vi "ZyklussteuerungGV_ECD.vi"(0 "Traps/MachKoeff0":dbl[](array[numeric]), 1 "DIOsNummern":cluster{"DIOsMod2BNr":i32[]}[](array[cluster]), 2 "error in":errorcluster, 5 "Traps/MachKoeff1":dbl[](array[numeric]), 7 "FPGA-VI-Referenz":refnum<k20>, 9 "Traps/MachKoeff2":dbl[](array[numeric]), 11 "Schieberegister":T1, 12 "Zeitpunkte/Setpoints":T2) -> (4 "Schieberegister":T1, 8 "error out":errorcluster)   [LabVIEW 2017]
uses:
  GVZwangs.vi
  GVHeizenLH.vi
  GVZeitenZyklen.vi
  <vilib>/Utility/error.llb/Error Cluster From Error Code.vi
  <vilib>/rvi/errors/niLvFpgaAdjustHostInterfaceError.vi
  GVHorstSP.vi
  GVZwangsMPV.vi
  GVZwangsMPVPos.vi
  GVVentilposition.vi
  <vilib>/rvi/interface/nirviReadWriteControl/nirviReadWriteControl.xnode
  FPGA Bitfiles/HAGAR-VECD_FPGATarget_FPGA-ProgrammECD_WS++LmW9gGg.lvbitx
  FPGA-Programm_ECD.vi
  NiFpgaLv.dll
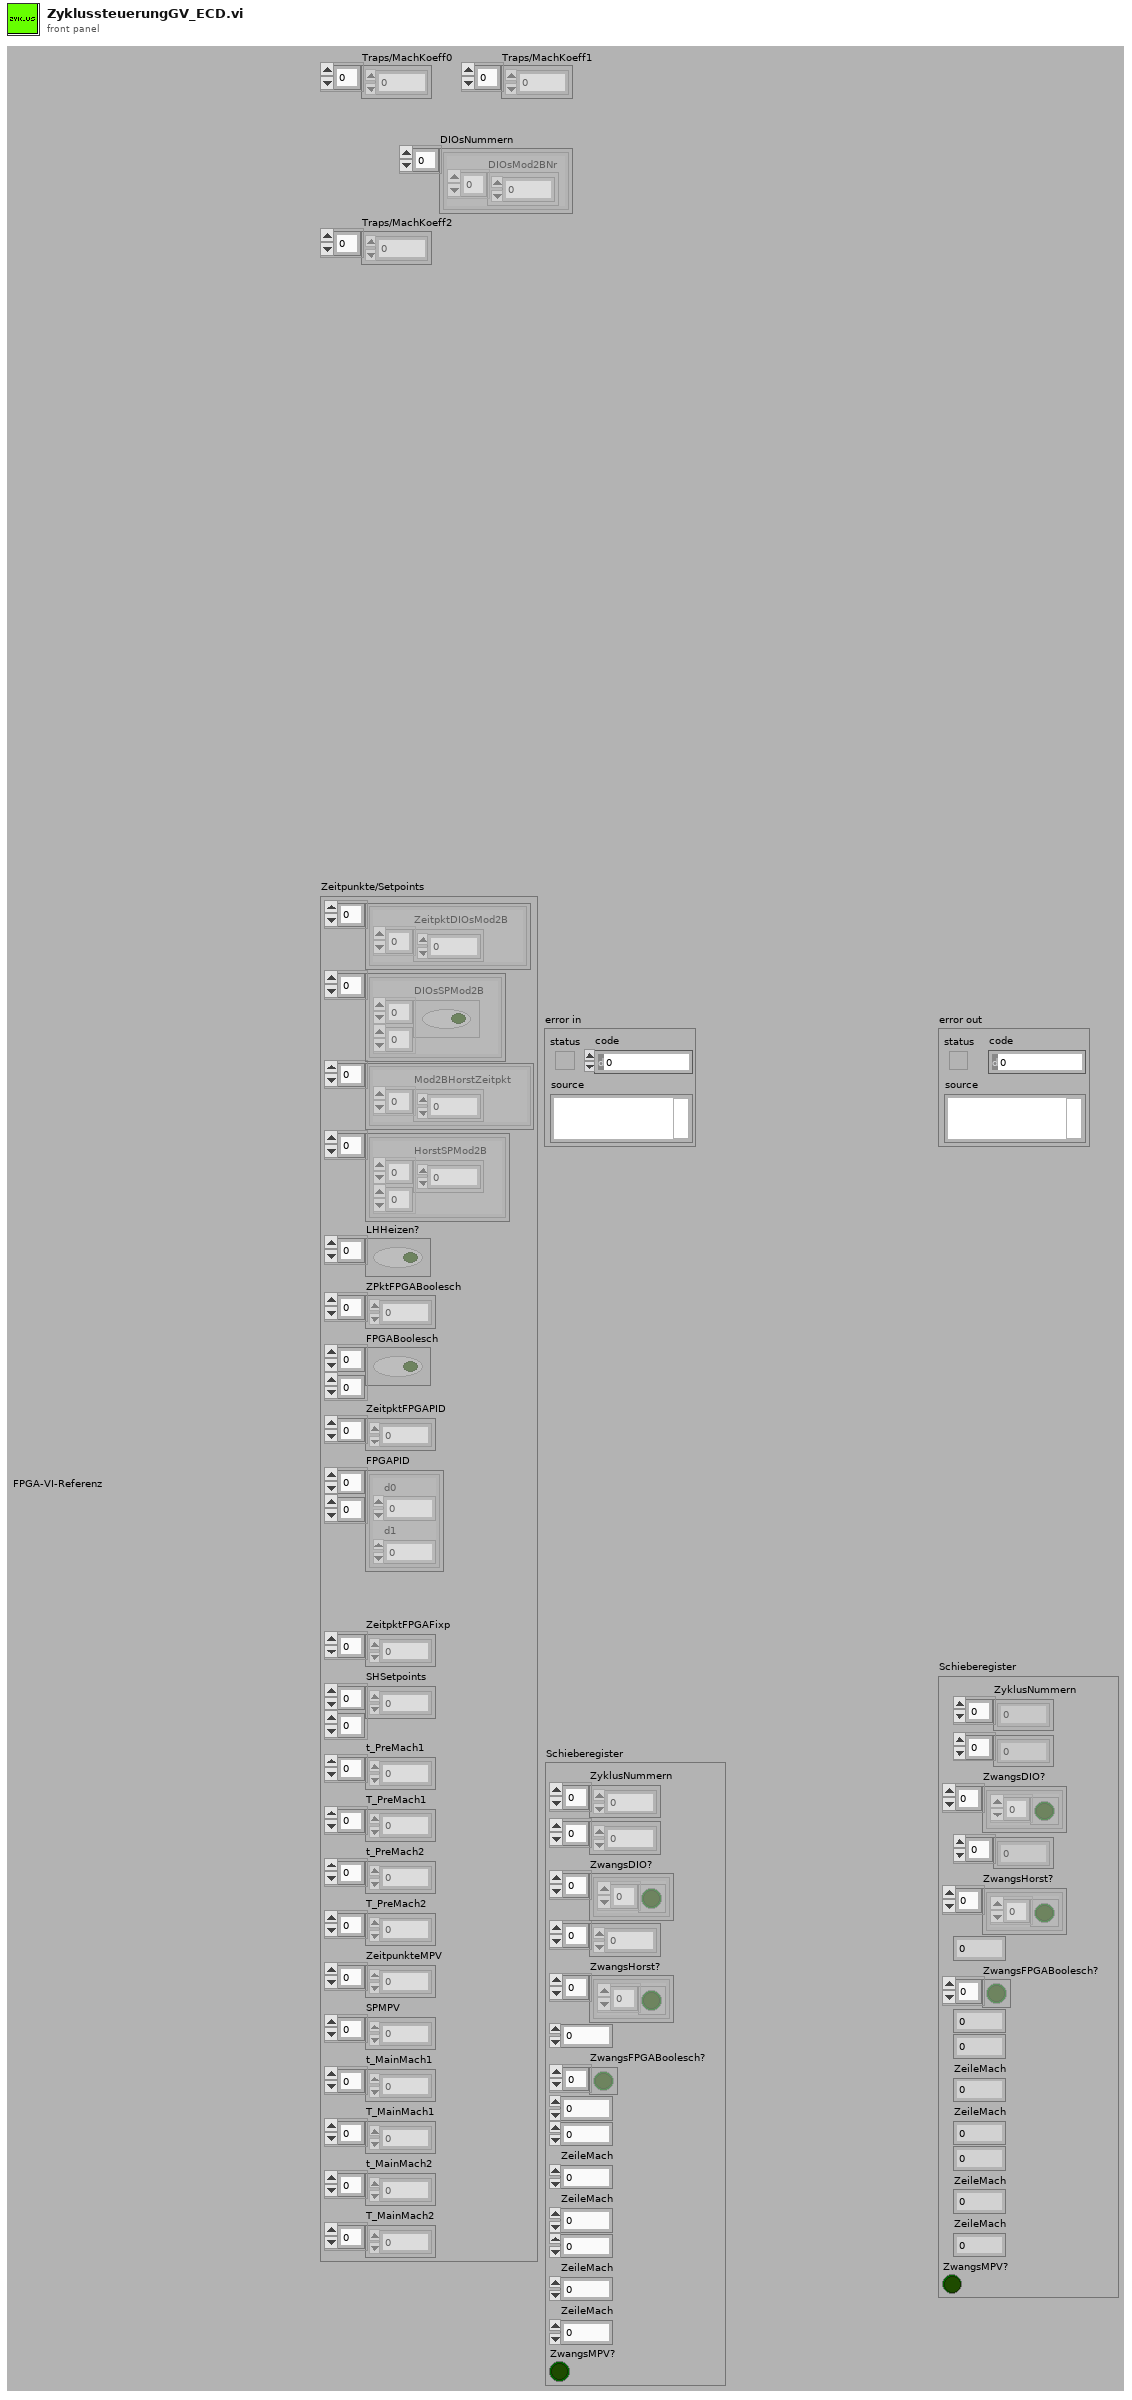
[diagram p1: front panel]
types:
  T1 = cluster{"ZyklusNummern":i32[], i32[], "ZwangsDIO?":cluster{bool[]}[], i32[], "ZwangsHorst?":cluster{bool[]}[], i32, "ZwangsFPGABoolesch?":bool[], i32, i32, "ZeileMach":i32, "ZeileMach":i32, i32, "ZeileMach":i32, "ZeileMach":i32, "ZwangsMPV?":bool}
  T2 = cluster{cluster{"ZeitpktDIOsMod2B":dbl[]}[], cluster{"DIOsSPMod2B":bool[][]}[], cluster{"Mod2BHorstZeitpkt":dbl[]}[], cluster{"HorstSPMod2B":dbl[][]}[], "LHHeizen?":bool[], "ZPktFPGABoolesch":dbl[], "FPGABoolesch":bool[][], "ZeitpktFPGAPID":dbl[], "FPGAPID":cluster{"d0":fxp<+/-,18,18>, "d1":fxp<+/-,21,21>}[][], "ZeitpktFPGAFixp":dbl[], "SHSetpoints":dbl[][], "t_PreMach1":dbl[], "T_PreMach1":dbl[], "t_PreMach2":dbl[], "T_PreMach2":dbl[], "ZeitpunkteMPV":dbl[], "SPMPV":i32[], "t_MainMach1":dbl[], "T_MainMach1":dbl[], "t_MainMach2":dbl[], "T_MainMach2":dbl[]}
  T3 = cluster{"d0":fxp<+/-,18,18>, "d1":fxp<+/-,21,21>}[][]
  T4 = cluster{"[0]":bool, "[1]":bool, "[2]":bool, "[3]":bool, "[4]":bool, "[5]":bool, "[6]":bool, "[7]":bool, "[8]":bool, "[9]":bool, "[10]":bool, "[11]":bool, "[12]":bool, "[13]":bool, "[14]":bool, "[15]":bool, "[16]":bool, "[17]":bool, "[18]":bool, "[19]":bool, "[20]":bool, "[21]":bool, "[22]":bool, "[23]":bool, "[24]":bool, "[25]":bool, "[26]":bool, "[27]":bool, "[28]":bool, "[29]":bool, "[30]":bool, "[31]":bool}
  T5 = cluster{"[0]":bool, "[1]":bool, "[2]":bool, "[3]":bool, "[4]":bool, "[5]":bool}
  T6 = cluster{"d0":fxp<+/-,18,18>, "d1":fxp<+/-,21,21>}[]
  T7 = cluster{"FPGAPID[0]":cluster{"d0":fxp<+/-,18,18>, "d1":fxp<+/-,21,21>}, "FPGAPID[1]":cluster{"d0":fxp<+/-,18,18>, "d1":fxp<+/-,21,21>}, "FPGAPID[2]":cluster{"d0":fxp<+/-,18,18>, "d1":fxp<+/-,21,21>}, "FPGAPID[3]":cluster{"d0":fxp<+/-,18,18>, "d1":fxp<+/-,21,21>}, "FPGAPID[4]":cluster{"d0":fxp<+/-,18,18>, "d1":fxp<+/-,21,21>}, "FPGAPID[5]":cluster{"d0":fxp<+/-,18,18>, "d1":fxp<+/-,21,21>}}
  T8 = cluster{"d0":fxp<+/-,18,18>, "d1":fxp<+/-,21,21>}
  T9 = cluster{"setpoint":fxp<+/-,26,5>, "setpoint":fxp<+/-,26,5>, "[2]":fxp<+/-,26,5>, "[3]":fxp<+/-,26,5>, "[4]":fxp<+/-,26,5>, "[5]":fxp<+/-,26,5>}
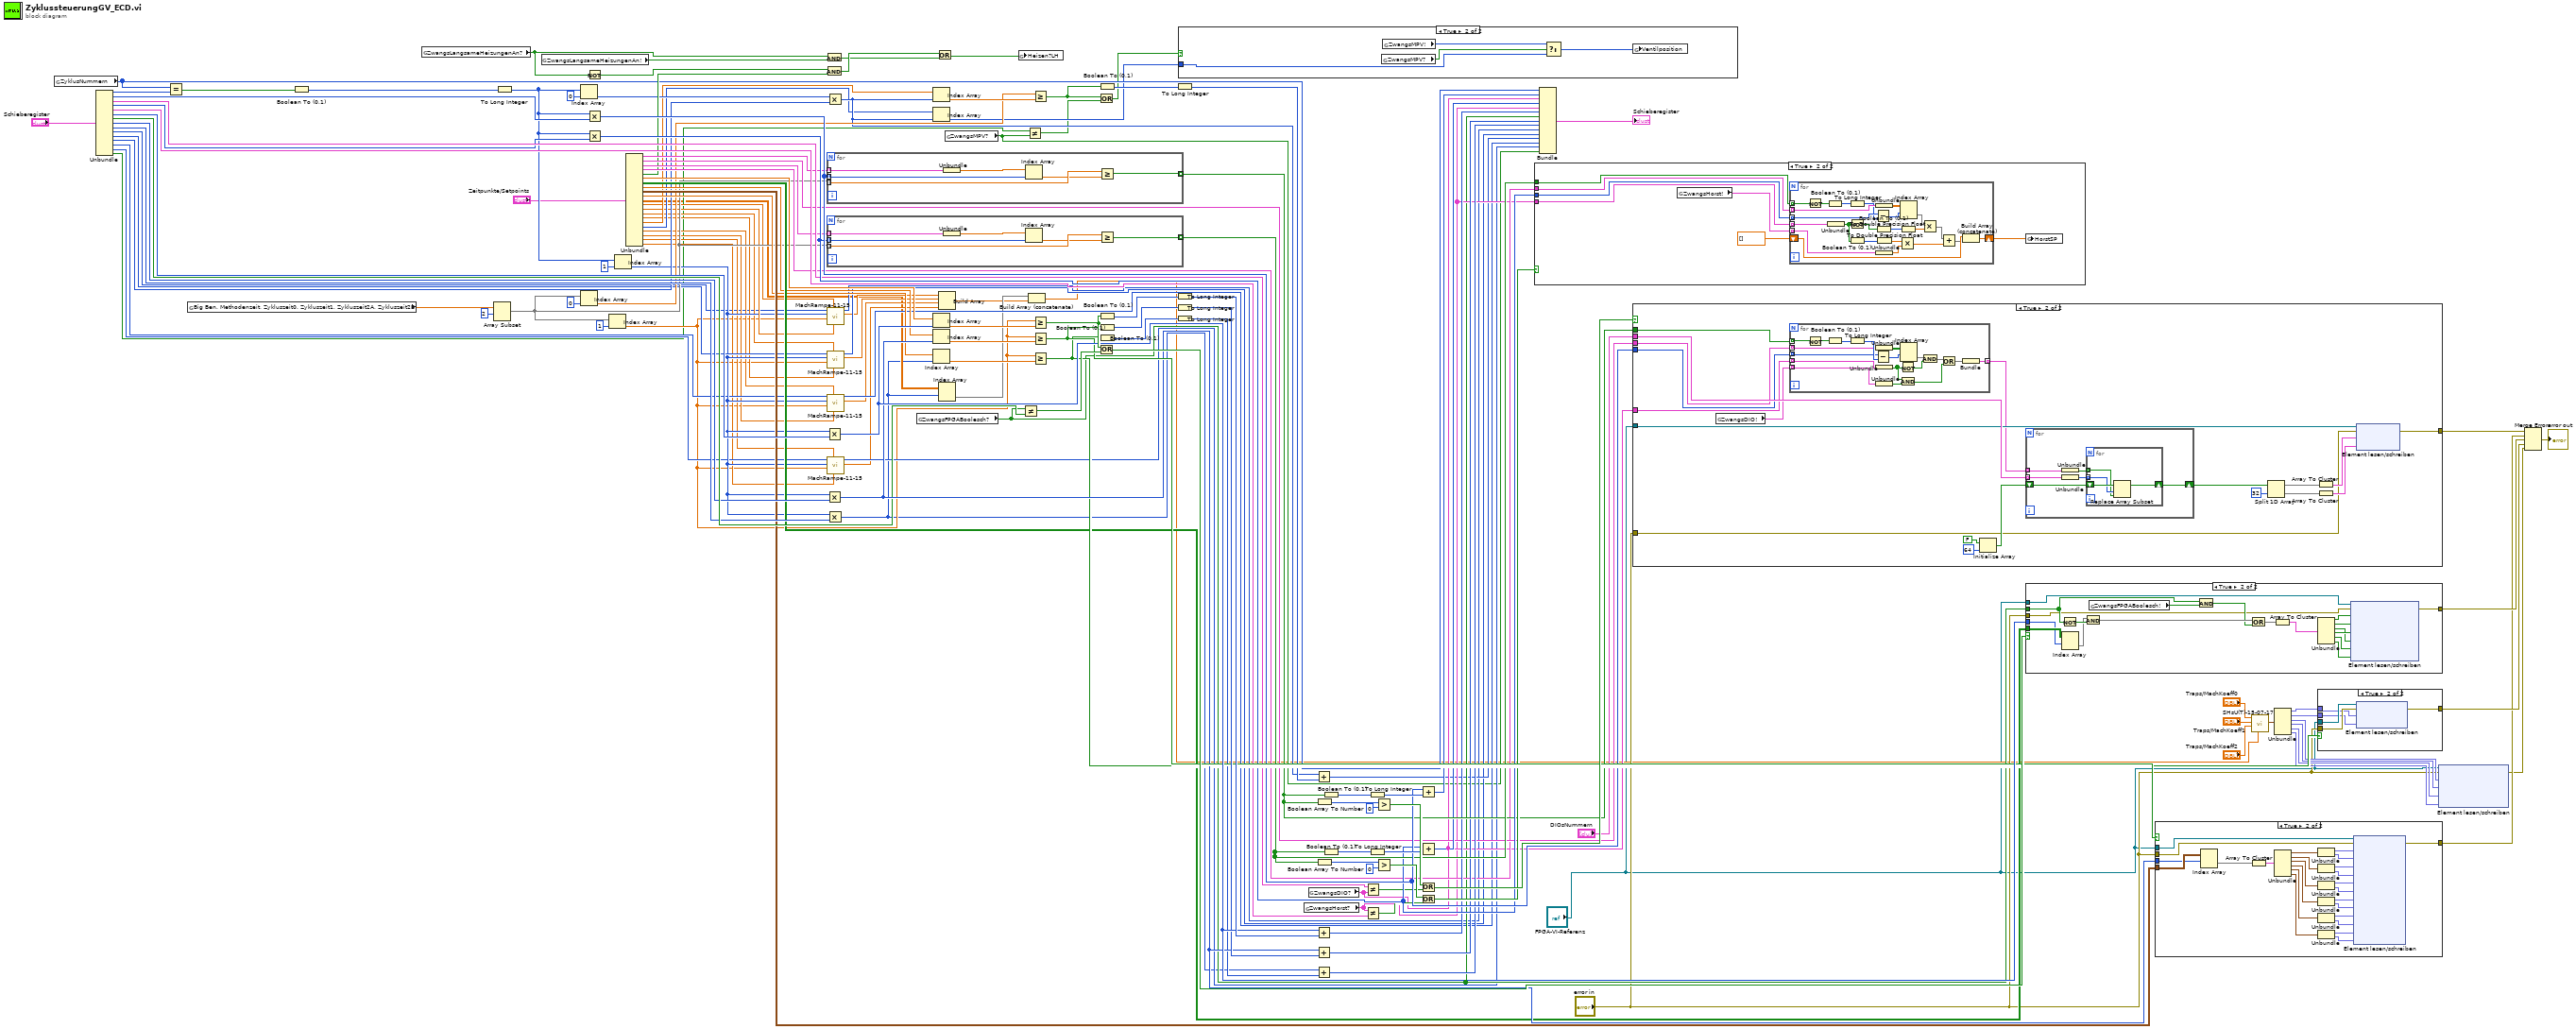
[diagram p0: block diagram]
diagram:
  n1 = global read "GVZeitenZyklen.vi" "ZyklusNummern"() -> (w58:i32[])
  n2 = Unbundle("Schieberegister") -> ("ZyklusNummern"=w101:i32[], w100:i32[], "ZwangsDIO?"=w99:cluster{bool[]}[], w98:i32[], "ZwangsHorst?"=w97:cluster{bool[]}[], w96:i32, "ZwangsFPGABoolesch?"=w95:bool[], w94:i32, w93:i32, "ZeileMach"=w35:i32, "ZeileMach"=w50:i32, w61:i32, "ZeileMach"=w48:i32, "ZeileMach"=w47:i32, "ZwangsMPV?"=w27:bool)
  n3 = Equal?(x=w58, y=w101) -> (x = y?=w143:bool[])
  n4 = global read "GVZeitenZyklen.vi" "Big Ben, Methodenzeit, Zykluszeit0, Zykluszeit1, Zykluszeit2A, Zykluszeit2B"() -> (w56:dbl[])
  n5 = Boolean To (0,1)(Boolean=w143) -> (0, 1=w142:i16[])
  n6 = global read "GVZwangs.vi" "ZwangsLangsameHeizungenAn?"() -> (w75:bool[])
  n7 = Array Subset(array=w56, index=2 ("Index")) -> (w55:dbl[])  [unwired: 1 in]
  n8 = To Long Integer(number=w142) -> (32bit integer=w71:i32[])
  n9 = global read "GVZwangs.vi" "ZwangsLangsameHeizungenAn!"() -> (w74:bool[])
  n10 = Index Array(array=w71, index=0 ("Index")) -> (element=w69:i32)
  n11 = Index Array(array=w55, index=0 ("Index")) -> (element=w66:dbl)
  n12 = Not(x=w75) -> (.not. x?=w112:bool[])
  n13 = Multiply(x=w71, y=w100) -> (x*y=w109:i32[])
  n14 = Multiply(x=w71, y=w98) -> (x*y=w106:i32[])
  n15 = Index Array(array=w55, index=1 ("Index")) -> (element=w36:dbl)
  n16 = Index Array(array=w71, index=1 ("Index")) -> (element=w49:i32)
  n17 = Unbundle("Zeitpunkte/Setpoints") -> (w87:cluster{"ZeitpktDIOsMod2B":dbl[]}[], w86:cluster{"DIOsSPMod2B":bool[][]}[], w85:cluster{"Mod2BHorstZeitpkt":dbl[]}[], w84:cluster{"HorstSPMod2B":dbl[][]}[], "LHHeizen?"=w83:bool[], "ZPktFPGABoolesch"=w82:dbl[], "FPGABoolesch"=w81:bool[][], "ZeitpktFPGAPID"=w80:dbl[], "FPGAPID"=w79:T3, "ZeitpktFPGAFixp"=w78:dbl[], "SHSetpoints"=w11:dbl[][], "t_PreMach1"=w53:dbl[], "T_PreMach1"=w52:dbl[], "t_PreMach2"=w46:dbl[], "T_PreMach2"=w45:dbl[], "ZeitpunkteMPV"=w60:dbl[], "SPMPV"=w59:i32[], "t_MainMach1"=w44:dbl[], "T_MainMach1"=w43:dbl[], "t_MainMach2"=w42:dbl[], "T_MainMach2"=w41:dbl[])
  n18 = And(x=w75, y=w74) -> (x .and. y?=w110:bool[])
  n19 = And(x=w112, y=w83) -> (x .and. y?=w111:bool[])
  n20 = Multiply(x=w49, y=w96) -> (x*y=w122:i32)
  n21 = Multiply(x=w49, y=w94) -> (x*y=w117:i32)
  n22 = Multiply(x=w69, y=w61) -> (x*y=w63:i32)
  n23 = for {
    tunnel: w109 -> [w149] mode=indexing
    tunnel: w55 -> [w148] mode=indexing
    tunnel: [w147] -> w103 mode=indexing
    tunnel: w87 -> [w145] mode=indexing
    n24 = Unbundle(w145) -> ("ZeitpktDIOsMod2B"=w144:dbl[])
    n25 = Index Array(array=w144, index=w149) -> (element=w146:dbl)
    n26 = Greater Or Equal?(x=w148, y=w146) -> (x >= y?=w147:bool)
  }
  n27 = for {
    tunnel: w106 -> [w155] mode=indexing
    tunnel: w55 -> [w154] mode=indexing
    tunnel: w85 -> [w151] mode=indexing
    tunnel: [w152] -> w107 mode=indexing
    n28 = Unbundle(w151) -> ("Mod2BHorstZeitpkt"=w150:dbl[])
    n29 = Index Array(array=w150, index=w155) -> (element=w153:dbl)
    n30 = Greater Or Equal?(x=w154, y=w153) -> (x >= y?=w152:bool)
  }
  n31 = call "MachRampe-11-15.vi"("T_Mach"=w52, "t_Mach"=w53, "ZykluszeitMod1"=w36, "gleicherZyklus?"=w49, "ZeileMach"=w35) -> ("T_Mach"=w34:dbl, "ZeileMach"=w51:i32)  [unwired: 5 in]
  n32 = call "MachRampe-11-15.vi"("T_Mach"=w45, "t_Mach"=w46, "ZykluszeitMod1"=w36, "gleicherZyklus?"=w49, "ZeileMach"=w50) -> ("T_Mach"=w33:dbl, "ZeileMach"=w40:i32)  [unwired: 5 in]
  n33 = call "MachRampe-11-15.vi"("T_Mach"=w43, "t_Mach"=w44, "ZykluszeitMod1"=w36, "gleicherZyklus?"=w49, "ZeileMach"=w48) -> ("T_Mach"=w32:dbl, "ZeileMach"=w39:i32)  [unwired: 5 in]
  n34 = call "MachRampe-11-15.vi"("T_Mach"=w41, "t_Mach"=w42, "ZykluszeitMod1"=w36, "gleicherZyklus?"=w49, "ZeileMach"=w47) -> ("T_Mach"=w31:dbl, "ZeileMach"=w38:i32)  [unwired: 5 in]
  n35 = Multiply(x=w49, y=w93) -> (x*y=w10:i32)
  n36 = global read "GVZwangs.vi" "ZwangsFPGABoolesch?"() -> (w72:bool[])
  n37 = Index Array(array=w60, index=w63) -> (element=w67:dbl)
  n38 = Index Array(array=w59, index=w63) -> (element=w30:i32)
  n39 = Index Array(array=w82, index=w122) -> (element=w128:dbl)
  n40 = Index Array(array=w80, index=w117) -> (element=w121:dbl)
  n41 = Index Array(array=w78, index=w10) -> (element=w116:dbl)
  n42 = Or(x=w111, y=w110) -> (x .or. y?=w73:bool[])
  n43 = Build Array(w34, w33, w32, w31) -> (w9:dbl[])
  n44 = Index Array(array=w11, index (row)=w10) -> (element=w12:dbl[])  [unwired: 1 in]
  n45 = global read "GVZwangsMPV.vi" "ZwangsMPV?"() -> (w28:bool)
  n46 = global write "GVHeizenLH.vi" "Heizen?LH"(w73) -> ()
  n47 = Not Equal?(x=w72, y=w95) -> (x != y?=w124:bool)
  n48 = Not Equal?(x=w27, y=w28) -> (x != y?=w26:bool)
  n49 = Build Array (concatenate)(w12, w9) -> (w3:dbl[])
  n50 = Greater Or Equal?(x=w66, y=w67) -> (x >= y?=w25:bool)
  n51 = Greater Or Equal?(x=w36, y=w128) -> (x >= y?=w125:bool)
  n52 = Greater Or Equal?(x=w36, y=w121) -> (x >= y?=w118:bool)
  n53 = Greater Or Equal?(x=w36, y=w116) -> (x >= y?=w113:bool)
  n54 = Or(x=w25, y=w26) -> (x .or. y?=w24:bool)
  n55 = Or(x=w125, y=w124) -> (x .or. y?=w123:bool)
  n56 = Boolean To (0,1)(Boolean=w25) -> (0, 1=w65:i16)
  n57 = Boolean To (0,1)(Boolean=w125) -> (0, 1=w127:i16)
  n58 = Boolean To (0,1)(Boolean=w118) -> (0, 1=w120:i16)
  n59 = Boolean To (0,1)(Boolean=w113) -> (0, 1=w115:i16)
  n60 = To Long Integer(number=w65) -> (32bit integer=w64:i32)
  n61 = To Long Integer(number=w127) -> (32bit integer=w126:i32)
  n62 = To Long Integer(number=w120) -> (32bit integer=w119:i32)
  n63 = To Long Integer(number=w115) -> (32bit integer=w114:i32)
  n64 = case shown="True" w24 {
    tunnel: w30 -> [_ w157]
    frame False {
    }
    frame True {
      n65 = global read "GVZwangsMPV.vi" "ZwangsMPV?"() -> (w159:bool)
      n66 = global read "GVZwangsMPVPos.vi" "ZwangsMPV!"() -> (w158:i32)
      n67 = Select(t=w158, s=w159, f=w157) -> (s? t:f=w156:i32)
      n68 = global write "GVVentilposition.vi" "Ventilposition"(w156) -> ()
    }
  }
  n69 = global read "GVZwangs.vi" "ZwangsHorst?"() -> (w76:cluster{bool[]}[])
  n70 = global read "GVZwangs.vi" "ZwangsDIO?"() -> (w77:cluster{bool[]}[])
  n71 = Add(x=w63, y=w64) -> (x+y=w62:i32)
  n72 = Add(x=w122, y=w126) -> (x+y=w90:i32)
  n73 = Add(x=w117, y=w119) -> (x+y=w89:i32)
  n74 = Add(x=w10, y=w114) -> (x+y=w88:i32)
  n75 = Boolean Array To Number(Boolean array=w103) -> (number=w139:u32)
  n76 = Boolean Array To Number(Boolean array=w107) -> (number=w133:u32)
  n77 = Boolean To (0,1)(Boolean=w103) -> (0, 1=w141:i16[])
  n78 = Boolean To (0,1)(Boolean=w107) -> (0, 1=w135:i16[])
  n79 = Not Equal?(x=w99, y=w77) -> (x != y?=w104:bool)
  n80 = Not Equal?(x=w76, y=w97) -> (x != y?=w105:bool)
  n81 = To Long Integer(number=w141) -> (32bit integer=w140:i32[])
  n82 = To Long Integer(number=w135) -> (32bit integer=w134:i32[])
  n83 = Greater?(x=w139, y=u32 0) -> (0:w136:bool)
  n84 = Greater?(x=w133, y=u32 0) -> (0:w131:bool)
  n85 = Add(x=w109, y=w140) -> (x+y=w92:i32[])
  n86 = Add(x=w106, y=w134) -> (x+y=w91:i32[])
  n87 = Or(x=w136, y=w104) -> (x .or. y?=w137:bool)
  n88 = Or(x=w131, y=w105) -> (x .or. y?=w108:bool)
  n89 = case shown="True" w108 {
    tunnel: w84 -> [_ w163]
    tunnel: w76 -> [_ w164]
    tunnel: w107 -> [_ w166]
    tunnel: w106 -> [_ w165]
    frame False {
    }
    frame True {
      n90 = global read "GVZwangs.vi" "ZwangsHorst!"() -> (w161:cluster{dbl[]}[])
      n91 = for {
        tunnel: w166 -> [w186] mode=indexing
        tunnel: w165 -> [w183] mode=indexing
        tunnel: w164 -> [w189] mode=indexing
        tunnel: w163 -> [w187] mode=indexing
        tunnel: w161 -> [w188] mode=indexing
        shift-right: [w167] -> w160
        shift-left: dbl[] [] -> [w169]
        n92 = Not(x=w186) -> (.not. x?=w185:bool)
        n93 = Boolean To (0,1)(Boolean=w185) -> (0, 1=w184:i16)
        n94 = Unbundle(w189) -> (w176:bool[])
        n95 = To Long Integer(number=w184) -> (32bit integer=w182:i32)
        n96 = Not(x=w176) -> (.not. x?=w179:bool[])
        n97 = Boolean To (0,1)(Boolean=w176) -> (0, 1=w177:i16[])
        n98 = Subtract(x=w183, y=w182) -> (x-y=w180:i32)
        n99 = Boolean To (0,1)(Boolean=w179) -> (0, 1=w178:i16[])
        n100 = Unbundle(w187) -> ("HorstSPMod2B"=w181:dbl[][])
        n101 = To Double Precision Float(number=w177) -> (double precision float=w173:dbl[])
        n102 = Unbundle(w188) -> (w172:dbl[])
        n103 = Multiply(x=w173, y=w172) -> (x*y=w170:dbl[])
        n104 = Index Array(array=w181, index (row)=w180) -> (element=w175:dbl[])  [unwired: 1 in]
        n105 = To Double Precision Float(number=w178) -> (double precision float=w174:dbl[])
        n106 = Multiply(x=w175, y=w174) -> (x*y=w171:dbl[])
        n107 = Add(x=w171, y=w170) -> (x+y=w168:dbl[])
        n108 = Build Array (concatenate)(w169, w168) -> (w167:dbl[])
      }
      n109 = global write "GVHorstSP.vi" "HorstSP"(w160) -> ()
    }
  }
  n110 = Bundle("ZyklusNummern"=w58, w92, "ZwangsDIO?"=w77, w91, "ZwangsHorst?"=w76, w90, "ZwangsFPGABoolesch?"=w72, w89, w88, "ZeileMach"=w51, "ZeileMach"=w40, w62, "ZeileMach"=w39, "ZeileMach"=w38, "ZwangsMPV?"=w28) -> (→"Schieberegister":T1)  [unwired: 1 in]
  n111 = case shown="True" w137 {
    tunnel: w109 -> [_ w205]
    tunnel: w77 -> [_ w202]
    tunnel: "DIOsNummern" -> [_ w209]
    tunnel: "FPGA-VI-Referenz" -> [_ w208]
    tunnel: w86 -> [_ w203]
    tunnel: w103 -> [_ w204]
    tunnel: "error in" -> [w190 w192]
    tunnel: [w190 w191] -> w19
    frame False {
    }
    frame True {
      n112 = global read "GVZwangs.vi" "ZwangsDIO!"() -> (w193:cluster{bool[]}[])
      n113 = for {
        tunnel: w205 -> [w224] mode=indexing
        tunnel: w204 -> [w223] mode=indexing
        tunnel: w203 -> [w222] mode=indexing
        tunnel: w202 -> [w221] mode=indexing
        tunnel: w193 -> [w220] mode=indexing
        tunnel: [w210] -> w201 mode=indexing
        n114 = Not(x=w223) -> (.not. x?=w226:bool)
        n115 = Boolean To (0,1)(Boolean=w226) -> (0, 1=w225:i16)
        n116 = To Long Integer(number=w225) -> (32bit integer=w227:i32)
        n117 = Subtract(x=w224, y=w227) -> (x-y=w218:i32)
        n118 = Unbundle(w222) -> ("DIOsSPMod2B"=w219:bool[][])
        n119 = Unbundle(w221) -> (w215:bool[])
        n120 = Unbundle(w220) -> (w214:bool[])
        n121 = Not(x=w215) -> (.not. x?=w216:bool[])
        n122 = And(x=w215, y=w214) -> (x .and. y?=w212:bool[])
        n123 = Index Array(array=w219, index (row)=w218) -> (element=w217:bool[])  [unwired: 1 in]
        n124 = And(x=w217, y=w216) -> (x .and. y?=w213:bool[])
        n125 = Or(x=w213, y=w212) -> (x .or. y?=w211:bool[])
        n126 = Bundle(w211) -> (w210:cluster{bool[]})  [unwired: 1 in]
      }
      n127 = Initialize Array(FALSE, 64 ("Dimension")) -> (w194:bool[])
      n128 = for {
        tunnel: w201 -> [w229] mode=indexing
        tunnel: w209 -> [w231] mode=indexing
        shift-right: [w232] -> w206
        shift-left: w194 -> [w233]
        n129 = Unbundle(w229) -> (w228:bool[])
        n130 = Unbundle(w231) -> ("DIOsMod2BNr"=w230:i32[])
        n131 = for {
          tunnel: w228 -> [w235] mode=indexing
          tunnel: w230 -> [w236] mode=indexing
          shift-right: [w234] -> w232
          shift-left: w233 -> [w237]
          n132 = Replace Array Subset(array=w237, new element=w235, index=w236) -> (w234:bool[])
        }
      }
      n133 = Split 1D Array(array=w206, index=32 ("Länge")) -> (first subarray=w200:bool[], second subarray=w198:bool[])
      n134 = Array To Cluster(array=w200) -> (cluster=w199:T4)
      n135 = Array To Cluster(array=w198) -> (cluster=w197:T4)
      n136 = xnode "Element lesen/schreiben"("FPGA-VI-Referenz (Eingang)"=w208, "Fehler (Eingang)"=w192, "Mod5/DIOs"=w199, "Mod6/DIOs"=w197) -> ("Fehler (Ausgang)"=w191:errorcluster)  [unwired: 1 out]
    }
  }
  n137 = case shown="True" w123 {
    tunnel: w122 -> [_ w248]
    tunnel: w72 -> [_ w253]
    tunnel: w81 -> [_ w257]
    tunnel: "FPGA-VI-Referenz" -> [_ w250]
    tunnel: "error in" -> [w238 w246]
    tunnel: [w238 w245] -> w22
    frame False {
    }
    frame True {
      n138 = Not(x=w253) -> (.not. x?=w256:bool[])
      n139 = Index Array(array=w257, index (row)=w248) -> (element=w255:bool[])  [unwired: 1 in]
      n140 = And(x=w255, y=w256) -> (x .and. y?=w254:bool[])
      n141 = global read "GVZwangs.vi" "ZwangsFPGABoolesch!"() -> (w247:bool[])
      n142 = And(x=w253, y=w247) -> (x .and. y?=w252:bool[])
      n143 = Or(x=w254, y=w252) -> (x .or. y?=w251:bool[])
      n144 = Array To Cluster(array=w251) -> (cluster=w249:T5)
      n145 = Unbundle(w249) -> ("[0]"=w244:bool, "[1]"=w243:bool, "[2]"=w242:bool, "[3]"=w241:bool, "[4]"=w240:bool, "[5]"=w239:bool)
      n146 = xnode "Element lesen/schreiben"("FPGA-VI-Referenz (Eingang)"=w250, "Fehler (Eingang)"=w246, "Heizen?Trap1"=w244, "Heizen?Trap2"=w243, "Heizen?PreMach1"=w242, "Heizen?PreMach2"=w241, "Heizen?MainMach1"=w240, "Heizen?MainMach2"=w239) -> ("Fehler (Ausgang)"=w245:errorcluster)  [unwired: 1 out]
    }
  }
  n147 = case shown="True" w118 {
    tunnel: "FPGA-VI-Referenz" -> [_ w283]
    tunnel: w79 -> [_ w282]
    tunnel: w117 -> [_ w279]
    tunnel: "error in" -> [w258 w278]
    tunnel: [w258 w277] -> w21
    frame False {
    }
    frame True {
      n148 = Index Array(array=w282, index (row)=w279) -> (element=w281:T6)  [unwired: 1 in]
      n149 = Array To Cluster(array=w281) -> (cluster=w280:T7)
      n150 = Unbundle(w280) -> ("FPGAPID[0]"=w276:T8, "FPGAPID[1]"=w273:T8, "FPGAPID[2]"=w270:T8, "FPGAPID[3]"=w267:T8, "FPGAPID[4]"=w264:T8, "FPGAPID[5]"=w261:T8)
      n151 = Unbundle(w276) -> ("d0"=w275:fxp<+/-,18,18>, "d1"=w274:fxp<+/-,21,21>)
      n152 = Unbundle(w273) -> ("d0"=w272:fxp<+/-,18,18>, "d1"=w271:fxp<+/-,21,21>)
      n153 = Unbundle(w270) -> ("d0"=w269:fxp<+/-,18,18>, "d1"=w268:fxp<+/-,21,21>)
      n154 = Unbundle(w267) -> ("d0"=w266:fxp<+/-,18,18>, "d1"=w265:fxp<+/-,21,21>)
      n155 = Unbundle(w264) -> ("d0"=w263:fxp<+/-,18,18>, "d1"=w262:fxp<+/-,21,21>)
      n156 = Unbundle(w261) -> ("d0"=w260:fxp<+/-,18,18>, "d1"=w259:fxp<+/-,21,21>)
      n157 = xnode "Element lesen/schreiben"("FPGA-VI-Referenz (Eingang)"=w283, "Fehler (Eingang)"=w278, "d0Trap1"=w275, "d1Trap1"=w274, "d0Trap2"=w272, "d1Trap2"=w271, "d0PreMach1"=w269, "d1PreMach1"=w268, "d0PreMach2"=w266, "d1PreMach2"=w265, "d0MainMach1"=w263, "d1MainMach1"=w262, "d0MainMach2"=w260, "d1MainMach2"=w259) -> ("Fehler (Ausgang)"=w277:errorcluster)  [unwired: 1 out]
    }
  }
  n158 = call "SHsU(T)-15-07-17.vi"("TemperaturenSH[V]"=w3, "Traps/MachKoeff2"="Traps/MachKoeff2", "Traps/MachKoeff1"="Traps/MachKoeff1", "Traps/MachKoeff0"="Traps/MachKoeff0") -> ("SpannungenSH"=w2:T9)  [unwired: 7 in]
  n159 = Unbundle(w2) -> ("setpoint"=w8:fxp<+/-,26,5>, "setpoint"=w7:fxp<+/-,26,5>, "[2]"=w18:fxp<+/-,26,5>, "[3]"=w17:fxp<+/-,26,5>, "[4]"=w16:fxp<+/-,26,5>, "[5]"=w15:fxp<+/-,26,5>)
  n160 = case shown="True" w113 {
    tunnel: "FPGA-VI-Referenz" -> [_ w289]
    tunnel: "error in" -> [w284 w288]
    tunnel: [w284 w287] -> w23
    tunnel: w8 -> [_ w286]
    tunnel: w7 -> [_ w285]
    frame False {
    }
    frame True {
      n161 = xnode "Element lesen/schreiben"("FPGA-VI-Referenz (Eingang)"=w289, "Fehler (Eingang)"=w288, "SetpointTrap1"=w286, "SetpointTrap2"=w285) -> ("Fehler (Ausgang)"=w287:errorcluster)  [unwired: 1 out]
    }
  }
  n162 = xnode "Element lesen/schreiben"("FPGA-VI-Referenz (Eingang)"="FPGA-VI-Referenz", "Fehler (Eingang)"="error in", "USetp[V]PreMach1"=w18, "USetp[V]PreMach2"=w17, "USetp[V]MainMach1"=w16, "USetp[V]MainMach2"=w15) -> ("Fehler (Ausgang)"=w13:errorcluster)  [unwired: 1 out]
  n163 = Merge Errors(w19, w21, w22, w23, w13) -> (→"error out":errorcluster)
